vi "WavelengthScanWithTimestamps.vi"(5 "error in (no error)":errorcluster, 6 "End wavelength":u16=1 min=1 step=1, 7 "Start wavelength":u16=1 min=1 step=1, 8 "VISA resource name":refnum<visa-resource-name>) -> (0 "error out":errorcluster, 1 "End time, s":dbl format="%#_9g", 2 "Start time, s":dbl format="%#_9g", 3 "VISA Refnum out":refnum<visa-resource-name>, 4 "Scan duration, s":dbl format="%#_9g")   [LabVIEW 2017, in "Spectral Products CM110.lvlib"]
uses:
  <vilib>/Instr/_visa.llb/Select Event Type.ctl
  Spectral Products CM110.lvlib
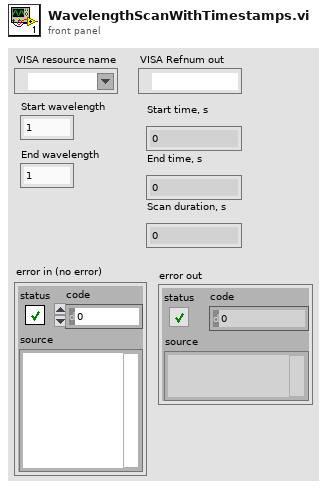
[diagram p1: front panel]
types:
  T1 = typedef "Select Event Type.ctl" = u32
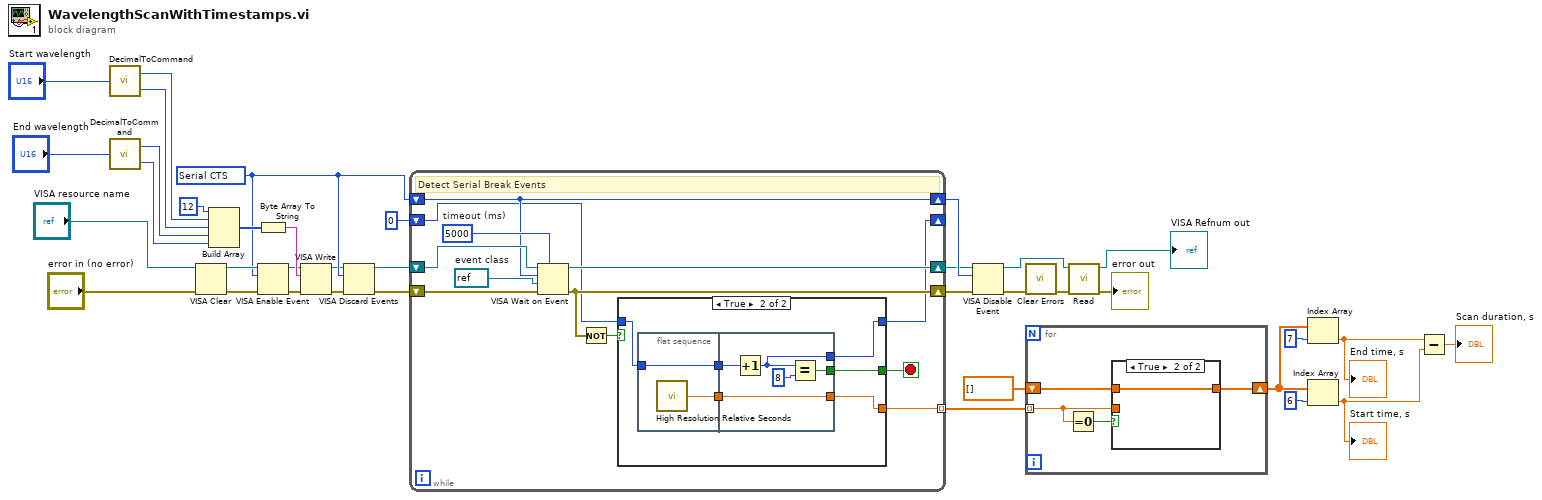
[diagram p0: block diagram]
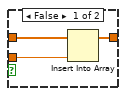
[diagram p2: hidden frame]
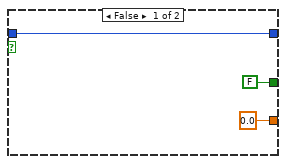
[diagram p3: hidden frame]
diagram:
  w21 = T1 1073684521 items=["Service Request"=1073684491, "Trigger"=3221168138, "Clear"=1073684493, "VXI Signal"=1073684512, "VXI/VME Interrupt"=3221168161, "VXI/VME Sysfail"=1073684509, "VXI/VME Sysreset"=1073684510, "GPIB CIC"=1073684498, "GPIB Talk"=1073684499, "GPIB Listen"=1073684500, "PXI Interrupt"=1073684514, "Serial Break"=1073684515, "Serial TermChar"=1073684516, "Serial CTS"=1073684521, "Serial DSR"=1073684522, "Serial DCD"=1073684524, "Serial RI"=1073684526, "Serial Character"=1073684533, "USB Interrupt"=1073684535, "All Enabled"=1073709055] ("Event Type")
  n1 = call "DecimalToCommand.vi"("Decimal"="Start wavelength") -> ("HiByte"=w35:u8, "LoByte"=w34:u8)  [unwired: 4 in]
  n2 = call "DecimalToCommand.vi"("Decimal"="End wavelength") -> ("HiByte"=w30:u8, "LoByte"=w29:u8)  [unwired: 4 in]
  n3 = VISA Clear(VISA resource name="VISA resource name", error in (no error)="error in (no error)") -> (VISA resource name out=w26:refnum<visa-resource-name>, error out=w25:errorcluster)
  n4 = Build Array(u8 12, w35, w34, w30, w29) -> (w33:u8[])
  n5 = Byte Array To String(unsigned byte array=w33) -> (string=w32:string)
  n6 = VISA Enable Event(8:w25, 10:w21, 11:w26) -> (0:w15:errorcluster, 3:w16:refnum<visa-resource-name>)  [unwired: 1 in]
  n7 = VISA Write(VISA resource name=w16, write buffer=w32, error in (no error)=w15) -> (VISA resource name out=w20:refnum<visa-resource-name>, error out=w19:errorcluster)  [unwired: 1 out]
  n8 = VISA Discard Events(8:w19, 10:w21, 11:w20) -> (0:w17:errorcluster, 3:w18:refnum<visa-resource-name>)  [unwired: 1 out]
  n9 = while {
    shift-right: [w44] -> w22
    shift-left: w18 -> [w48]
    tunnel: [w45] -> w14 mode=indexing
    shift-right: [w43] -> w24
    shift-left: w17 -> [w46]
    shift-right: [w47] -> w23
    shift-left: w21 -> [w47]
    shift-right: [w38] -> _
    shift-left: 0 -> [w40]
    stop <- w39 stop-if-true
    w42 = refnum<visa-resource-name> refnum  # event class
    w49 = u32 5000  # timeout (ms)
    # "Detect Serial Break Events"
    n10 = VISA Wait on Event(7:w49, 8:w46, 9:w42, 10:w47, 11:w48) -> (0:w43:errorcluster, 3:w44:refnum<visa-resource-name>)  [unwired: 2 out]
    n11 = Not(x=w43) -> (.not. x?=w41:bool)
    n12 = case shown="True" w41 {
      tunnel: [0.0 ("relative seconds") w58] -> w45
      tunnel: w40 -> [w50 w55]
      tunnel: [FALSE w54] -> w39
      tunnel: [w50 w53] -> w38
      frame False {
      }
      frame True {
        n13 = flat-sequence {
          tunnel: [w60] -> w57
          tunnel: [w59] -> w56
          tunnel: w55 -> [w59]
          tunnel: [w65] -> w58
          tunnel: w57 -> [w65]
          tunnel: w56 -> [w64]
          tunnel: [w62] -> w54
          tunnel: [w61] -> w53
          frame #0 {
            n14 = call <vilib>:"High Resolution Relative Seconds.vi"() -> ("relative seconds"=w60:dbl)
          }
          frame #1 {
            n15 = Increment(x=w64) -> (x+1=w61:i32)
            n16 = Equal?(x=w61, y=8) -> (x = y?=w62:bool)
          }
        }
      }
    }
  }
  n17 = VISA Disable Event(8:w24, 10:w23, 11:w22) -> (0:w11:errorcluster, 3:w4:refnum<visa-resource-name>)  [unwired: 1 out]
  n18 = call <vilib>:"Clear Errors.vi"("error in (no error)"=w11) -> ("error out"=w3:errorcluster)  [unwired: 5 in, 1 out]
  n19 = for {
    tunnel: w14 -> [w67] mode=indexing
    shift-right: [w66] -> w7
    shift-left: dbl[] [] -> [w68]
    n20 = Equal To 0?(x=w67) -> (x = 0?=w69:bool)
    n21 = case shown="True" w69 {
      tunnel: w68 -> [w72 w73]
      tunnel: w67 -> [w71 _]
      tunnel: [w70 w73] -> w66
      frame False {
        n22 = Insert Into Array(array=w72, new element=w71) -> (w70:dbl[])  [unwired: 1 in]
      }
      frame True {
      }
    }
  }
  n23 = call "Read.vi"("error in (no error)"=w3, "VISA Refnum in"=w4) -> ("error out"=→"error out":errorcluster, "VISA Refnum out"=→"VISA Refnum out":refnum<visa-resource-name>)  [unwired: 6 in, 2 out]
  n24 = Index Array(array=w7, index=7) -> (element=w6:dbl)
  "End time, s" <- w6
  n25 = Index Array(array=w7, index=6) -> (element=w5:dbl)
  "Start time, s" <- w5
  n26 = Subtract(x=w6, y=w5) -> (x-y=→"Scan duration, s":dbl)
